vi "Send Error Messages.vi"(8 "error in (no error)":errorcluster) -> (0 "error out":errorcluster)   [LabVIEW 2023, in "Encoder.lvlib"]
uses:
  Encoder.lvlib
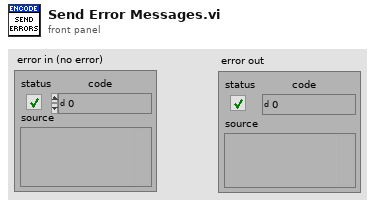
[diagram p1: front panel]
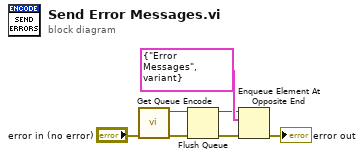
[diagram p0: block diagram]
diagram:
  n1 = call "Get Queue Encode.vi"("error in (no error)"="error in (no error)") -> ("error out"=w4:errorcluster, "Decoder Queue"=w3:refnum<queue>)  [unwired: 9 in]
  n2 = Flush Queue(queue=w3, error in (no error)=w4) -> (queue out=w1:refnum<queue>, error out=w2:errorcluster)  [unwired: 1 out]
  n3 = Enqueue Element At Opposite End(queue=w1, element=cluster{string, variant} {"Error Messages", variant}, error in (no error)=w2) -> (error out=→"error out":errorcluster)  [unwired: 1 in, 2 out]
